vi "RTM - Apply Tx Configuration.vi"(8 "error in (no error)":errorcluster, 11 "Node Ptr":T1 format="%.0x") -> (0 "error out":errorcluster)   [LabVIEW 2016, in "UDP-Custom-Device System Explorer.lvlib"]
uses:
  UDP-Custom-Device System Explorer.lvlib
  <vilib>/NI Veristand/Custom Device API/Custom Device Item Ref.ctl
  <vilib>/NI VeriStand/Custom Device API/Custom Device API.lvlib
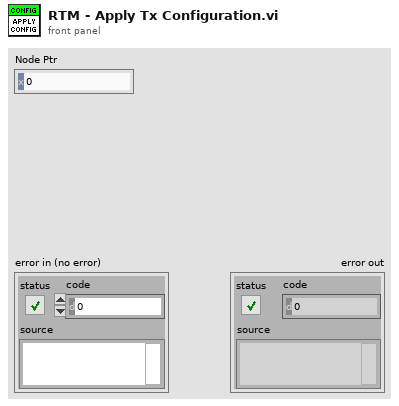
[diagram p1: front panel]
types:
  T1 = typedef "Custom Device API.lvlib/Custom Device Item Ref.ctl" = u64
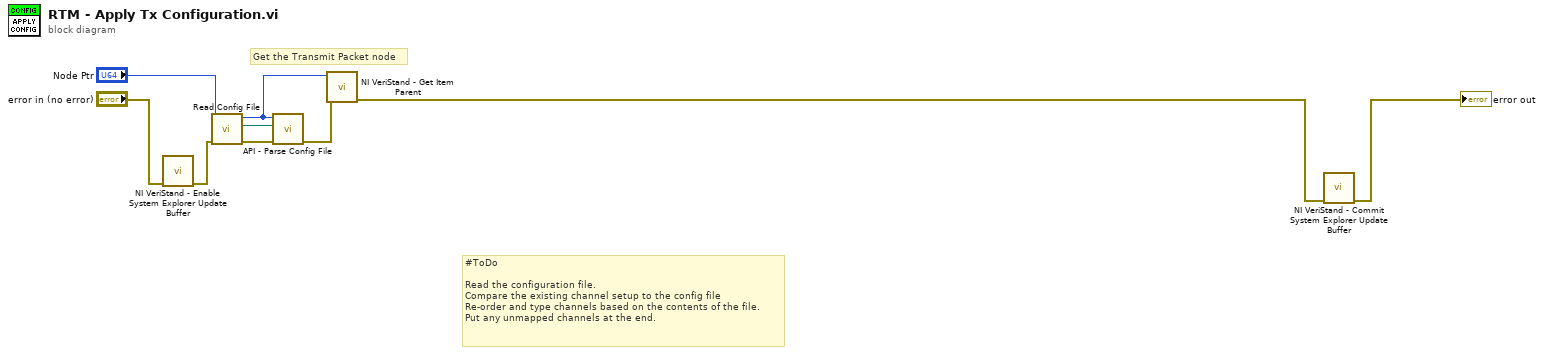
[diagram p0: block diagram]
diagram:
  # "#ToDo\n\nRead the configuration file.\nCompare the existing channel setup to the config file\nRe-order and type channels based on the contents of the file.\nPut any unmapped channels at the end."
  # "Get the Transmit Packet node"
  n1 = call <vilib>:"NI VeriStand - Enable System Explorer Update Buffer.vi"("error in (no error)"="error in (no error)") -> ("error out"=w3:errorcluster)  [unwired: 10 in]
  n2 = call "Read Config File.vi"("error in (no error)"=w3, "Node Ptr"="Node Ptr") -> ("error out"=w8:errorcluster, "Config File"=w7:path, "Node Ptr out"=w9:T1)  [unwired: 7 in]
  n3 = call "API - Parse Config File.vi"("error in (no error)"=w8, "Config Path"=w7, "Node Ptr"=w9) -> ("error out"=w6:errorcluster)  [unwired: 6 in, 2 out]
  n4 = call <vilib>:"NI VeriStand - Get Item Parent.vi"("error in (no error)"=w6, "Item Ref in"=w9) -> ("error out"=w2:errorcluster)  [unwired: 6 in, 3 out]
  n5 = call <vilib>:"NI VeriStand - Commit System Explorer Update Buffer.vi"("error in (no error)"=w2) -> ("error out"=→"error out":errorcluster)  [unwired: 10 in]
